vi "Save File Bus File.vi"(8 "Error In":errorcluster, 11 "Debug File Path":path) -> (0 "Error Out":errorcluster, 3 "Bus Path":path)   [LabVIEW 2016, in "Save File.lvlib"]
uses:
  Save File.lvlib
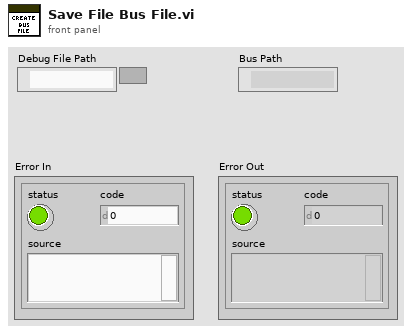
[diagram p1: front panel]
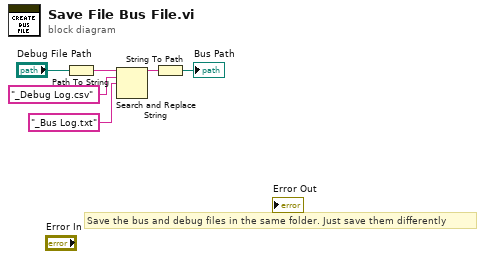
[diagram p0: block diagram]
diagram:
  # "Save the bus and debug files in the same folder. Just save them differently"
  n1 = Path To String(path="Debug File Path") -> (string=w4:string)
  n2 = Search and Replace String(input string=w4, search string="_Debug Log.csv" ("Debug"), replace string="_Bus Log.txt" ("replace string (\"\")")) -> (result string=w2:string)  [unwired: 5 in, 3 out]
  n3 = String To Path(string=w2) -> (path=→"Bus Path":path)
